vi "Save.vi"() -> ()   [LabVIEW 2015]
panel:
  in  "Input Loop time (sec)":dbl
  out "Time (sec)":sgl
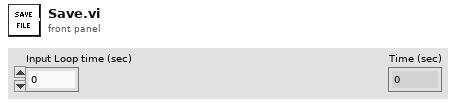
[diagram p1: front panel]
types:
  T1 = enum16{"open", "replace", "create", "open or create", "replace or create", "replace or create with confirmation"}
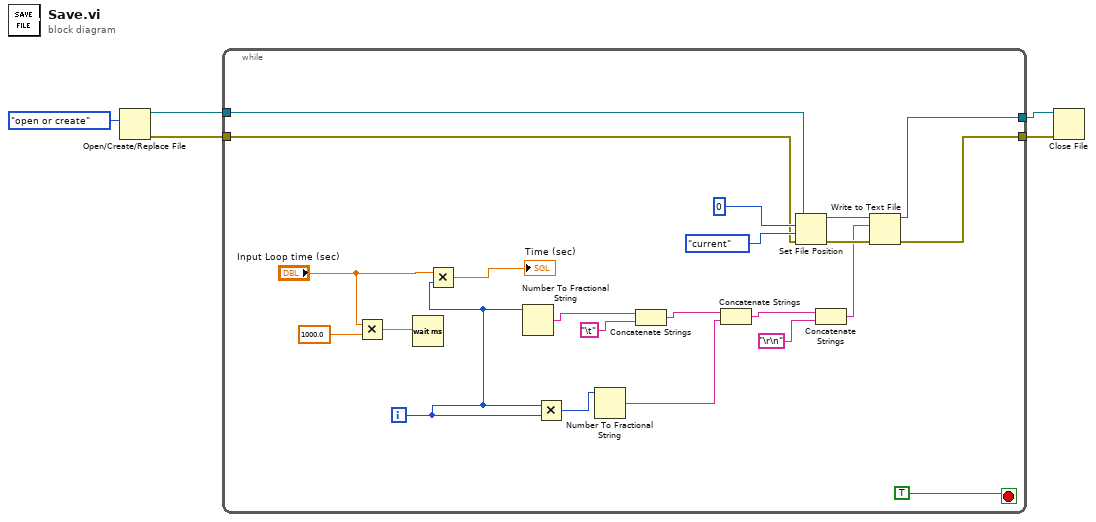
[diagram p0: block diagram]
diagram:
  n1 = Open/Create/Replace File(operation (0:open)=T1."open or create") -> (refnum out=w2:refnum<file>, error out=w4:errorcluster)  [unwired: 5 in, 1 out]
  n2 = while {
    tunnel: w4 -> [w8]
    tunnel: [w7] -> w3
    tunnel: w2 -> [w13]
    tunnel: [w9] -> w1
    i -> [w23]
    stop <- TRUE ("Boolean") stop-if-true
    n3 = Multiply(x="Input Loop time (sec)", y=1000.0) -> (x*y=w26:dbl)
    n4 = Wait (ms)(milliseconds to wait=w26) -> ()  [unwired: 1 out]
    n5 = Multiply(x="Input Loop time (sec)", y=w23) -> (x*y=→"Time (sec)":dbl)
    n6 = Number To Fractional String(number=w23) -> (F-format string=w21:string)  [unwired: 3 in]
    n7 = Multiply(x=w23, y=w23) -> (x*y=w22:i32)
    n8 = Number To Fractional String(number=w22) -> (F-format string=w19:string)  [unwired: 3 in]
    n9 = Concatenate Strings(w21, "\t") -> (w18:string)
    n10 = Concatenate Strings(w18, w19) -> (w17:string)
    n11 = Set File Position(offset (in bytes) (0)=i64 0, refnum=w13, from (0:start)=enum16{"start", "end", "current"}."current", error in=w8) -> (refnum out=w12:refnum<file>, error out=w11:errorcluster)
    n12 = Concatenate Strings(w17, "\r\n") -> (w10:string)
    n13 = Write to Text File(file (use dialog)=w12, text=w10, error in=w11) -> (refnum out=w9:refnum<file>, error out=w7:errorcluster)  [unwired: 1 in, 1 out]
  }
  n14 = Close File(refnum=w1, error in=w3) -> ()  [unwired: 2 out]
